vi "Package Parameters for Asynch VIs.vi"(10 "cluster":T1={"Device Error"={"status"=FALSE, "code"=0, "source"=""}, "J1939 Process Parameters"={"J1939 XNET Settings"={"XNET Database"="", "XNET Cluster"="", "CAN Port"="", "Baud rate [Bd]"=0, "Termination"=0, "Incoming Rate"=0, "Outcoming Rate"=1, "Write Decimation"=1}, "Incoming Single Point Configuraiton"={"ID"=[], "Conversion"=[], "Channel Array Positions"=[], "Frame Length"=[]}, "Outgoing Cyclic Configuraiton"={"ID"=[], "Conversion"=[], "Channel Array Positions"=[], "Frame Length"=[], "Transmit Propreties"=[]}, "J1939 Monitor Settings"={"J1939 Network Address"=0, "Name"=0}, "Simulated Addresses"=[], "Simulated Addresses LUT"=variant, "Name"=""}, "Internal Command Engine References"={"Name"="", "Response Refs"={"Values Array"=[], "Response Names"=[]}, "Command Refs"={"Values Array"=[], "Command Names"=[]}}, "FPGA Session"=0, "Incoming Decimation"=0, "Outgoing Decimation"=0, "Processes"=refnum} {"J1939 Process Parameters"."Simulated Addresses"."Simulated Addresses"."J1939 XNET Settings"."Name" format="%.0x"; "J1939 Process Parameters"."J1939 Monitor Settings"."Name" format="%.0x"; "J1939 Process Parameters"."Outgoing Cyclic Configuraiton"."Transmit Propreties"."Transmit Time" format="%#_p"; "J1939 Process Parameters"."J1939 XNET Settings"."Termination" items=["Off", "On"]}) -> (3 "Array":cluster{"VI":refnum<vi>, "Parameters":variant}[](array[cluster]))   [LabVIEW 2015, in "J1939 Addon Engine.lvlib"]
uses:
  J1939 Addon Engine.lvlib
  Types/Inline Device Cluster.ctl
  <vilib>/NI/NI VeriStand Inline Async API/_VS Inline Async API/VS Inline Async API/VS Inline Async API.lvclass
  Types/Process Parameters.ctl
  Shared/Types/XNET Settings.ctl
  Types/Incoming Single Point Configuration.ctl
  Types/Outgoing Cyclic Configuration.ctl
  Shared/Types/XNET Frame Event Properties.ctl
  Shared/Types/Monitor Settings.ctl
  Types/Simulated Settings.ctl
  Shared/Types/Compiled Simulated Settings.ctl
  <vilib>/NI Veristand/Custom Device API/Block Data Reference.ctl
  <vilib>/NI Veristand/Custom Device API/Data Reference.ctl
  Types/DTC FIFOs.ctl
  Shared/Types/SysDef Command Settings.ctl
  <vilib>/NI VeriStand/Custom Device API/Custom Device API.lvlib
  Shared/J1939 Addon Shared.lvlib
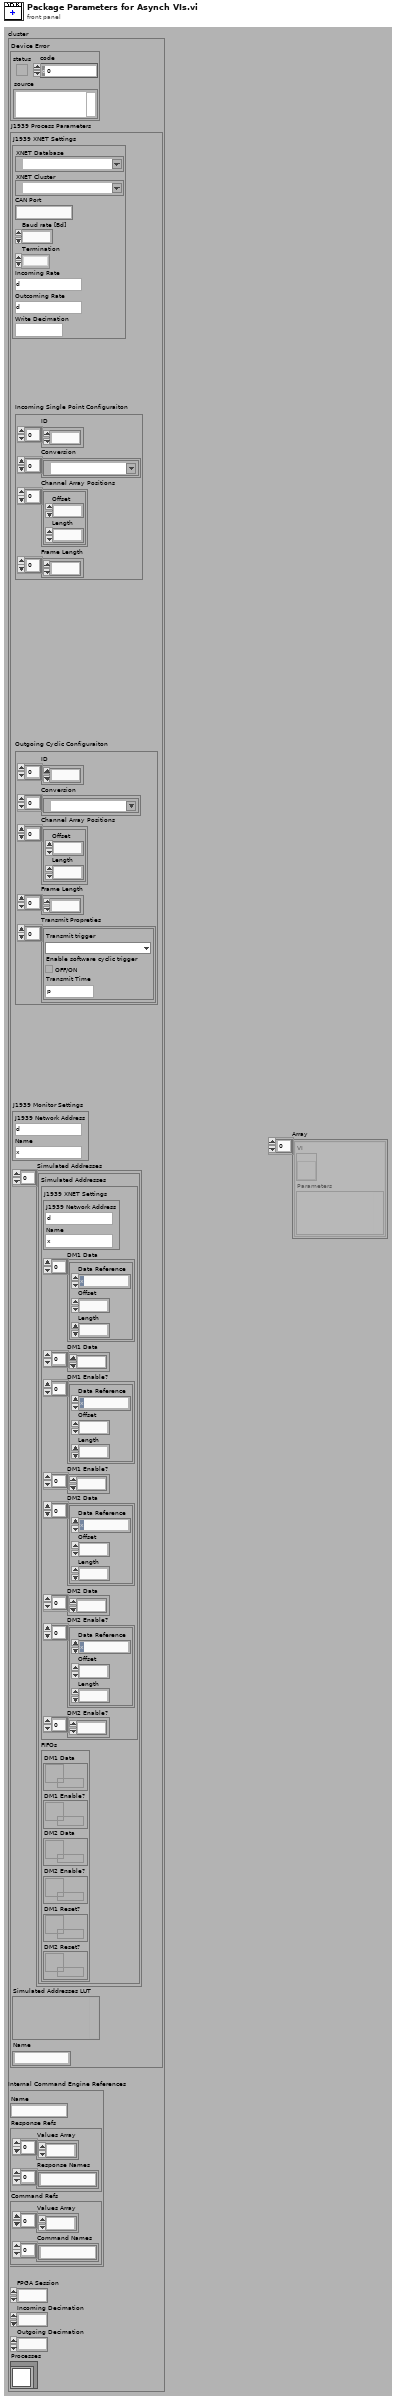
[diagram p1: front panel]
types:
  T1 = typedef "J1939 Addon Engine.lvlib/Inline Device Cluster.ctl" = cluster{"Device Error":errorcluster, "J1939 Process Parameters":T2, "Internal Command Engine References":T13, "FPGA Session":u32, "Incoming Decimation":u32, "Outgoing Decimation":u32, "Processes":refnum<class "VS Inline Async API.lvclass">}
  T2 = typedef "J1939 Addon Engine.lvlib/Process Parameters.ctl" = cluster{"J1939 XNET Settings":T3, "Incoming Single Point Configuraiton":T4, "Outgoing Cyclic Configuraiton":T5, "J1939 Monitor Settings":T7, "Simulated Addresses":T8[], "Simulated Addresses LUT":variant, "Name":string}
  T3 = typedef "J1939 Addon Shared.lvlib/XNET Settings.ctl" = cluster{"XNET Database":refnum<k21>, "XNET Cluster":refnum<k21>, "CAN Port":string, "Baud rate [Bd]":u32, "Termination":u32, "Incoming Rate":u32, "Outcoming Rate":u32, "Write Decimation":u32}
  T4 = typedef "J1939 Addon Engine.lvlib/Incoming Single Point Configuration.ctl" = cluster{"ID":u32[], "Conversion":refnum<k21>[], "Channel Array Positions":cluster{"Offset":u32, "Length":u32}[], "Frame Length":u32[]}
  T5 = typedef "J1939 Addon Engine.lvlib/Outgoing Cyclic Configuration.ctl" = cluster{"ID":u32[], "Conversion":refnum<k21>[], "Channel Array Positions":cluster{"Offset":u32, "Length":u32}[], "Frame Length":u32[], "Transmit Propreties":T6[]}
  T6 = typedef "J1939 Addon Shared.lvlib/XNET Frame Event Properties.ctl" = cluster{"Transmit trigger":enum16{"Channel value change"}, "Enable software cyclic trigger":bool, "Transmit Time":dbl}
  T7 = typedef "J1939 Addon Shared.lvlib/Monitor Settings.ctl" = cluster{"J1939 Network Address":u8, "Name":u64}
  T8 = typedef "J1939 Addon Engine.lvlib/Simulated Settings.ctl" = cluster{"Simulated Addresses":T9, "FIFOs":T12}
  T9 = typedef "J1939 Addon Shared.lvlib/Compiled Simulated Settings.ctl" = cluster{"J1939 XNET Settings":T7, "DM1 Data":T10[], "DM1 Data":dbl[], "DM1 Enable?":T10[], "DM1 Enable?":dbl[], "DM2 Data":T10[], "DM2 Data":dbl[], "DM2 Enable?":T10[], "DM2 Enable?":dbl[]}
  T10 = typedef "Custom Device API.lvlib/Block Data Reference.ctl" = cluster{"Data Reference":T11, "Offset":u64, "Length":u64}
  T11 = typedef "Custom Device API.lvlib/Data Reference.ctl" = i32
  T12 = typedef "J1939 Addon Engine.lvlib/DTC FIFOs.ctl" = cluster{"DM1 Data":refnum<k33>, "DM1 Enable?":refnum<k33>, "DM2 Data":refnum<k33>, "DM2 Enable?":refnum<k33>, "DM1 Reset?":refnum<k33>, "DM2 Reset?":refnum<k33>}
  T13 = typedef "J1939 Addon Shared.lvlib/SysDef Command Settings.ctl" = cluster{"Name":string, "Response Refs":cluster{"Values Array":dbl[], "Response Names":string[]}, "Command Refs":cluster{"Values Array":dbl[], "Command Names":string[]}}
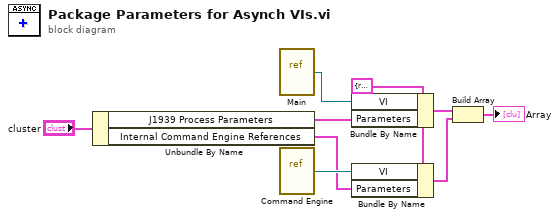
[diagram p0: block diagram]
diagram:
  w4 = cluster{"VI":refnum<vi>, "Parameters":variant} {"VI"=refnum, "Parameters"=variant} ("Process")
  n1 = Unbundle By Name("cluster") -> ("J1939 Process Parameters"=w7:T2, "Internal Command Engine References"=w5:T13)
  n2 = vi-ref "Main.vi"() -> (w8:refnum<vi>)
  n3 = vi-ref "Command Engine.vi"() -> (w6:refnum<vi>)
  n4 = Bundle By Name(cluster=w4, "VI"=w8, "Parameters"=w7) -> (w3:cluster{"VI":refnum<vi>, "Parameters":variant})
  n5 = Bundle By Name(cluster=w4, "VI"=w6, "Parameters"=w5) -> (w2:cluster{"VI":refnum<vi>, "Parameters":variant})
  n6 = Build Array(w3, w2) -> (→"Array":cluster{"VI":refnum<vi>, "Parameters":variant}[])
